vi "LocalVariable.vi"() -> ()   [LabVIEW 2022 SP3]
panel:
  in  "D":bool
  in  "C":bool
  in  "B":bool
  in  "A":bool
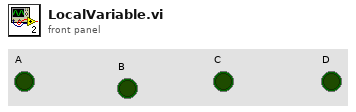
[diagram p1: front panel]
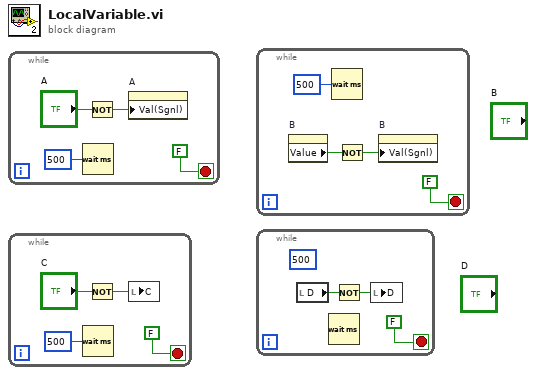
[diagram p0: block diagram]
diagram:
  n1 = while {
    stop <- FALSE stop-if-true
    n2 = Wait (ms)(milliseconds to wait=u32 500) -> ()  [unwired: 1 out]
    n3 = Not(x="A") -> (.not. x?=w1:bool)
    n4 = property on="A" class="Bool (strict)"("Val(Sgnl)"=w1) -> ()  [unwired: 2 in, 2 out]
  }
  n5 = while {
    stop <- FALSE stop-if-true
    n6 = Wait (ms)(milliseconds to wait=u32 500) -> ()  [unwired: 1 out]
    n7 = Not(x="C") -> (.not. x?=w5:bool)
    n8 = local write "C"(w5) -> ()
  }
  n9 = while {
    stop <- FALSE stop-if-true
    n10 = property on="B" class="Bool (strict)"() -> ("Value"=w9:bool)  [unwired: 2 in, 2 out]
    n11 = Wait (ms)(milliseconds to wait=u32 500) -> ()  [unwired: 1 out]
    n12 = Not(x=w9) -> (.not. x?=w10:bool)
    n13 = property on="B" class="Bool (strict)"("Val(Sgnl)"=w10) -> ()  [unwired: 2 in, 2 out]
  }
  n14 = while {
    stop <- FALSE stop-if-true
    (unwired) u32 500 ("milliseconds to wait")
    n15 = local read "D"() -> (w14:bool)
    n16 = Wait (ms)() -> ()  [unwired: 1 in, 1 out]
    n17 = Not(x=w14) -> (.not. x?=w13:bool)
    n18 = local write "D"(w13) -> ()
  }
